vi "WINAPI Is 64 Bit OS.vi"() -> (0 "error out":errorcluster, 3 "Is64Bit":bool)   [LabVIEW 2015, in "MiscHelperVIs.lvlib"]
uses:
  MiscHelperVIs.lvlib
  kernel32.dll
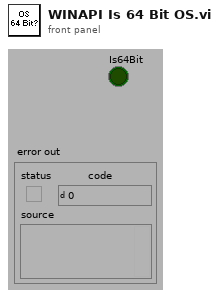
[diagram p1: front panel]
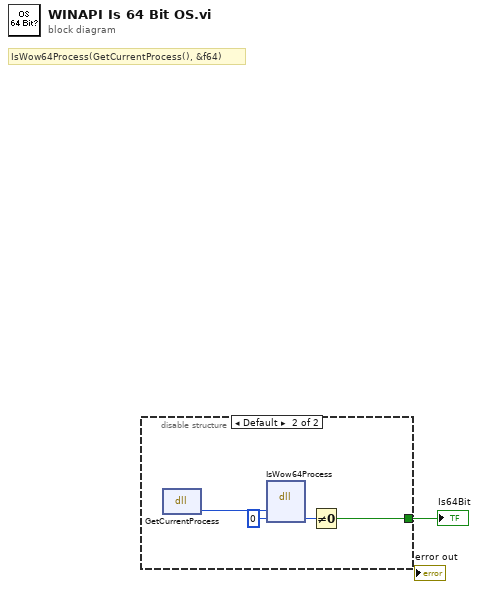
[diagram p0: block diagram]
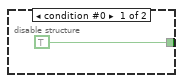
[diagram p2: hidden frame]
diagram:
  # "IsWow64Process(GetCurrentProcess(), &f64)"
  n1 = disable-structure shown="Default" {
    disable-tunnel: [TRUE w4] -> w1
    frame condition #0 {
    }
    frame condition #1 (active) {
      n2 = dll-call lib="kernel32.dll" fn="GetCurrentProcess"() -> ("return type"=w3:u64)  [unwired: 3 in, 2 out]
      n3 = dll-call lib="kernel32.dll" fn="IsWow64Process"("pid"=w3, "arg"=0) -> ("arg"=w5:u32)  [unwired: 5 in, 2 out]
      n4 = Not Equal To 0?(x=w5) -> (x != 0?=w4:bool)
    }
  }
  "Is64Bit" <- w1
